vi "Gantry_GUI.vi"(0 "COMPORT":refnum<visa-resource-name>="COM5", 5 "error in (no error)":errorcluster, 7 "Antenna Select":u16(ring) items=["HOME", "TX1", "TX2", "TX3", "TX4", "TX5", "TX6", "TX7", "TX8", "TX9", "TX10", "TX11", "TX12", "RX8", "RX7", "RX6", "RX5", "RX4", "RX3", "RX2", "RX1"], 8 "EnableDriver(t)":bool=TRUE, 9 "z ref":dbl=21.0 format="%#_6f", 10 "Operation":u16(ring) items=["W/R", "RD ONLY", "WR ONLY"], 11 "Set-Z(Inches)":dbl=21.0 format="%#_6f") -> (3 "Coordinates Ref File":path=path "C:/RageATE-Tetra/Instruments/Zaber Gantry/Labview Code from Colin/Gantry/antenna_cords-4.csv", 14 "GantryGuiRefOut":refnum<vi>, 19 "error out":errorcluster)   [LabVIEW 2018]
uses:
  Initialize References/Sequence Globals.vi
  <vilib>/Utility/file.llb/Read Delimited Spreadsheet (DBL).vi
panel:
  out "stripped path":path
  in  "Exe_write":bool
  in  "Exit":bool
  out "Success?(t)":bool
  in  "Exe_ctrl":bool
  in  "Set-zMach":dbl format="%#_6f"
  out "Get-z":dbl=21.0 format="%#_6f"
  out "Get-y":dbl format="%#_13g"
  out "Get-x":dbl
  out "py path":path=path "C:/RageATE-Tetra/Instruments/Zaber Gantry/Labview Code from Colin/Gantry/Gantry.py"
  in  "Selector Control":T1(radio)
  out "comport":string="COM5"
  in  "Close Serial(t)":bool
  in  "Set-y":dbl format="%#_13g"
  in  "Set-x":dbl
  out "begin":dbl=9735.3466752 format="%_19f"
  out "List":dbl[][](array[numeric])
  # "X-Y Controls"
  # "Z Controls"
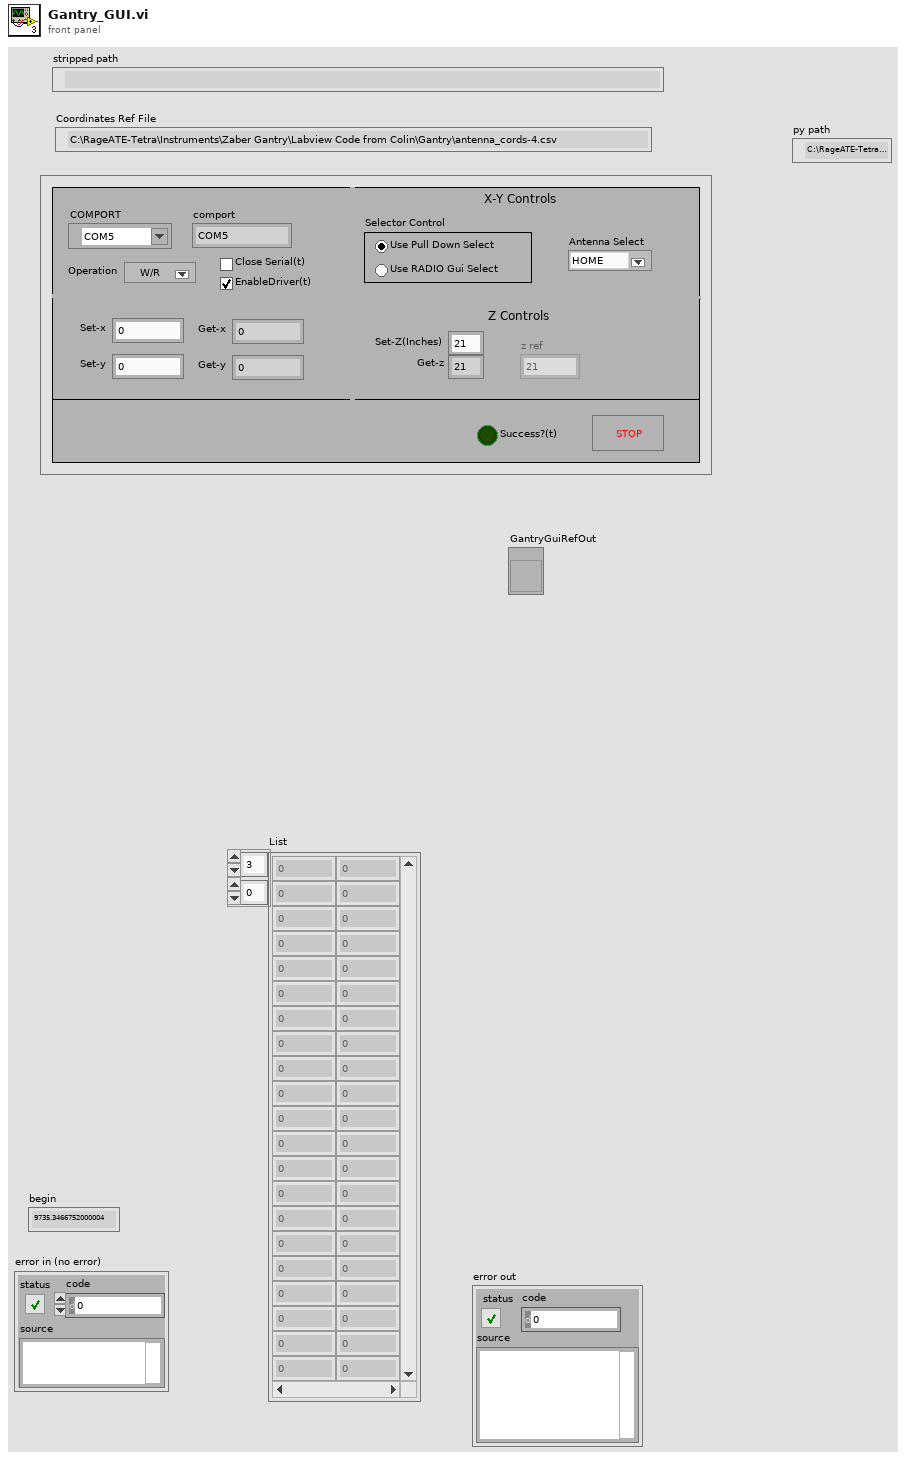
[diagram p1: front panel]
types:
  T1 = enum32{"Use Pull Down Select", "Use RADIO Gui Select"}
  T2 = enum32{"Invalid", "Standard", "Closed", "Hidden", "Minimized", "Maximized"}
  T3 = enum8{"Enabled", "Disabled", "Disabled and Grayed Out"}
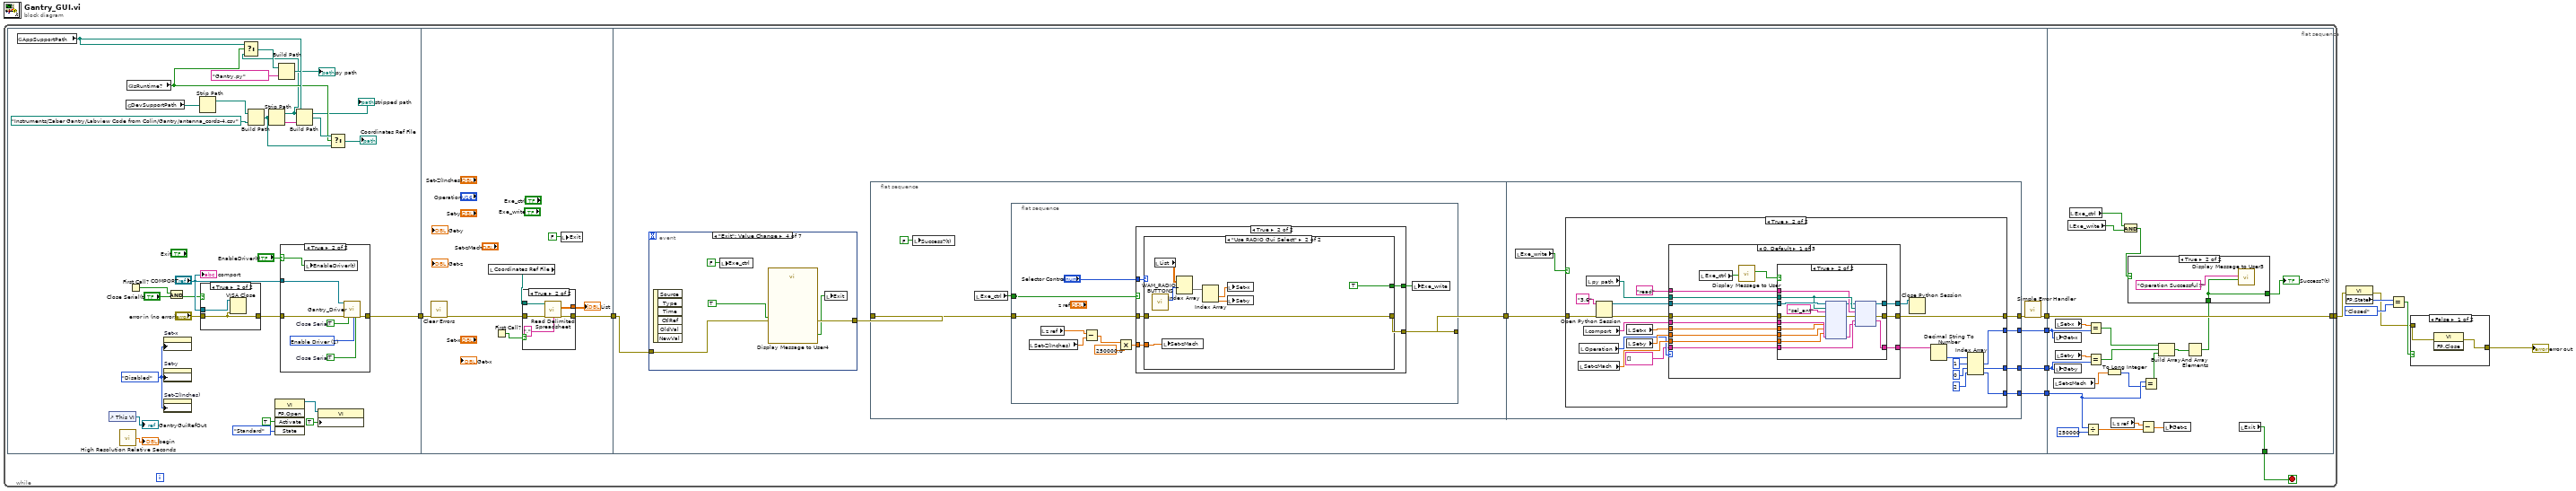
[diagram p0: block diagram]
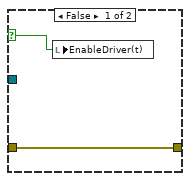
[diagram p4: hidden frame]
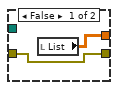
[diagram p5: hidden frame]
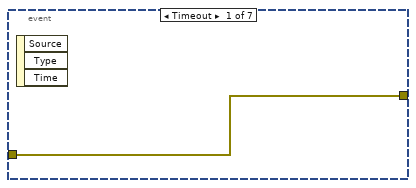
[diagram p6: hidden frame]
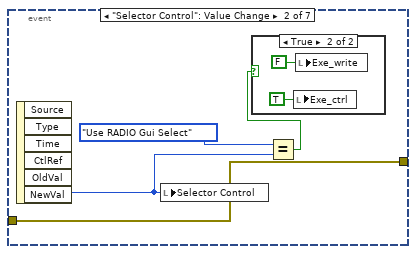
[diagram p7: hidden frame]
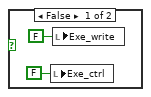
[diagram p8: hidden frame]
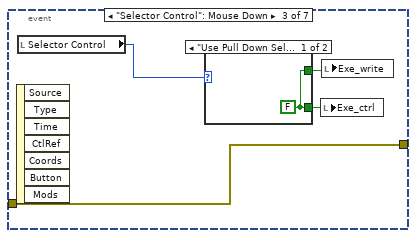
[diagram p9: hidden frame]
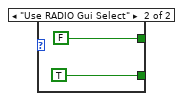
[diagram p10: hidden frame]
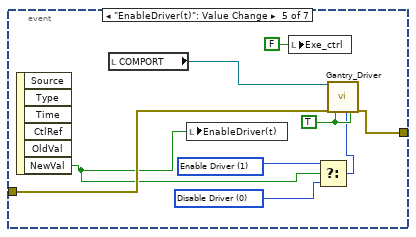
[diagram p11: hidden frame]
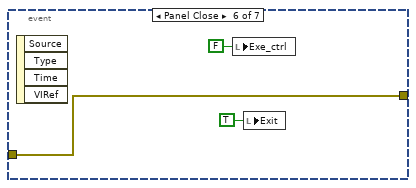
[diagram p12: hidden frame]
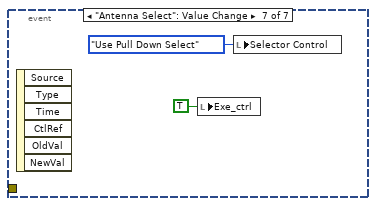
[diagram p13: hidden frame]
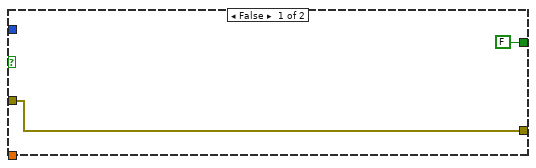
[diagram p14: hidden frame]
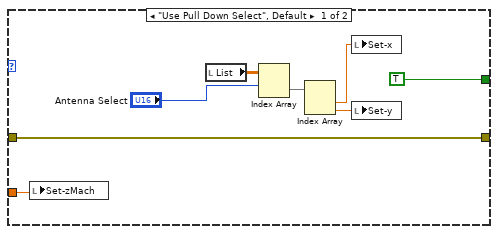
[diagram p15: hidden frame]
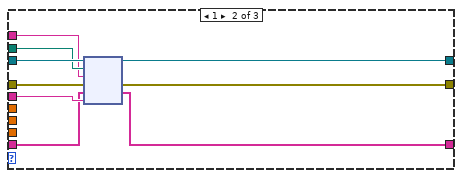
[diagram p18: hidden frame]
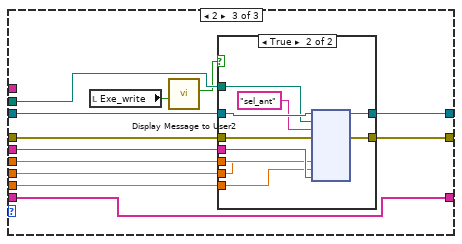
[diagram p19: hidden frame]
diagram:
  n1 = while {
    tunnel: [w8] -> w1
    stop <- w7 stop-if-true
    n2 = flat-sequence {
      tunnel: [w37] -> w14
      tunnel: w14 -> [w61]
      tunnel: [w58] -> w13
      tunnel: [w73] -> w12
      tunnel: [w76] -> w11
      tunnel: [w75] -> w10
      tunnel: [w72] -> w9
      tunnel: w13 -> [w69]
      tunnel: w12 -> [w264]
      tunnel: [w264] -> w8
      tunnel: w11 -> [w253]
      tunnel: w10 -> [w256]
      tunnel: w9 -> [w259]
      tunnel: [w248] -> w7
      frame #0 {
        w34 = T3."Disabled" ("Disabled")
        n3 = global read "Sequence Globals.vi" "AppSupportPath"() -> (w23:path)
        n4 = control-ref of="This VI"() -> (→"GantryGuiRefOut":refnum<vi>)
        n5 = call <vilib>:"High Resolution Relative Seconds.vi"() -> ("relative seconds"=→"begin":dbl)
        n6 = global read "Sequence Globals.vi" "DevSupportPath"() -> (w16:path)
        n7 = global read "Sequence Globals.vi" "IsRuntime?"() -> (w21:bool)
        n8 = First Call?() -> (First Call?: T/F=w32:bool)
        n9 = property on="Set-x" class="DigNum (strict)"("DisabledEnum"=w34) -> ()  [unwired: 2 in, 2 out]
        n10 = property on="Set-y" class="DigNum (strict)"("DisabledEnum"=w34) -> ()  [unwired: 2 in, 2 out]
        n11 = property on="Set-Z(Inches)" class="DigNum (strict)"("DisabledEnum"=w34) -> ()  [unwired: 2 in, 2 out]
        n12 = And(x=w32, y="Close Serial(t)") -> (x .and. y?=w33:bool)
        n13 = Strip Path(path=w16) -> (stripped path=w26:path)  [unwired: 1 out]
        n14 = case shown="True" w33 {
          tunnel: "error in (no error)" -> [w43 w44]
          tunnel: [w43 w44] -> w39
          tunnel: "COMPORT" -> [_ w45]
          frame False {
          }
          frame True {
            n15 = VISA Close(VISA resource name=w45, error in (no error)=w44) -> ()  [unwired: 1 out]
          }
        }
        n16 = Build Path(base path=w26, name or relative path=path "Instruments/Zaber Gantry/Labview Code from Colin/Gantry/antenna_cords-4.csv" ("file path (dialog if empty)")) -> (appended path=w25:path)
        n17 = Strip Path(path=w25) -> (stripped path=w15:path, name=w24:string)
        "stripped path" <- w15
        n18 = Select(t=w23, s=w21, f=w15) -> (s? t:f=w20:path)
        n19 = invoke class="VI" method="FP.Open"("Activate"=TRUE ("Activate?"), "State"=T2."Standard") -> (reference out=w29:refnum<vi>)  [unwired: 3 in, 4 out]
        n20 = Build Path(base path=w20, name or relative path="Gantry.py") -> (appended path=→"py path":path)
        n21 = case shown="True" "EnableDriver(t)" {
          selector: "EnableDriver(t)" -> [w46 w48]
          tunnel: "COMPORT" -> [_ w51]
          tunnel: w39 -> [w47 w54]
          tunnel: [w47 w50] -> w37
          frame False {
            n22 = local write "EnableDriver(t)"(w46) -> ()
          }
          frame True {
            w49 = TRUE  # Close Serial
            w52 = u16 1 items=["Disable Driver", "Enable Driver", "Read Driver Status"] ("Driver-Func")
            w53 = TRUE  # Close Serial
            n23 = local write "EnableDriver(t)"(w48) -> ()
            n24 = call "Gantry_Driver.vi"("VISA resource name"=w51, "error in (no error)"=w54, "Open Serial"=w53, "Driver-Func"=w52, "Close Serial"=w49) -> ("error out"=w50:errorcluster)  [unwired: 11 in, 3 out]
          }
        }
        n25 = Build Path(base path=w23, name or relative path=w24) -> (appended path=w22:path)
        n26 = property class="VI"(reference=w29, "Front Panel.IsFrontmost"=TRUE ("Front Panel Window:Is Frontmost")) -> ()  [unwired: 1 in, 2 out]
        n27 = Select(t=w22, s=w21, f=w25) -> (s? t:f=→"Coordinates Ref File":path)
        "comport" <- "COMPORT"
      }
      frame #1 {
        n28 = call <vilib>:"Clear Errors.vi"("error in (no error)"=w61) -> ("error out"=w60:errorcluster)  [unwired: 5 in, 1 out]
        n29 = local read "Coordinates Ref File"() -> (w55:path)
        n30 = First Call?() -> (First Call?: T/F=w57:bool)
        n31 = case shown="True" w57 {
          tunnel: w60 -> [w62 w68]
          tunnel: w55 -> [_ w67]
          tunnel: [w63 w65] -> w59
          tunnel: [w62 w64] -> w58
          frame False {
            n32 = local read "List"() -> (w63:dbl[][])
          }
          frame True {
            n33 = call-poly <vilib>:"Read Delimited Spreadsheet.vi"("file path (dialog if empty)"=w67, "error in (no error)"=w68, "delimiter (\\t)"="," ("delimiter (\\t)")) -> ("all rows"=w65:dbl[][], "error out"=w64:errorcluster)  [unwired: 7 in, 4 out]
          }
        }
        "List" <- w59
        n34 = local write "Exit"(FALSE ("Exit")) -> ()
      }
      frame #2 {
        n35 = event shown="[3] \"Exit\": Value Change" {
          selector: _ -> [_ _ _ _ _ _ _]
          dyn-events: _ -> [_ _ _ _ _ _ _]
          timeout: _ -> [_ _ _ _ _ _ _]
          tunnel: w69 -> [w77 w81 w89 w95 w105 w108 _]
          tunnel: [w77 w81 w89 w95 w104 w108 _] -> w70
          event Timeout {
            n36 = event-data() -> ()  [unwired: 1 in, 3 out]
          }
          event "Selector Control": Value Change {
            n37 = event-data() -> ("NewVal"=w80:T1)  [unwired: 1 in, 5 out]
            n38 = local write "Selector Control"(w80) -> ()
            n39 = Equal?(x=T1."Use RADIO Gui Select", y=w80) -> (x = y?=w78:bool)
            n40 = case shown="True" w78 {
              frame False {
                n41 = local write "Exe_ctrl"(FALSE ("Exe_ctrl")) -> ()
                n42 = local write "Exe_write"(FALSE ("Exe_write")) -> ()
              }
              frame True {
                n43 = local write "Exe_ctrl"(TRUE ("Exe_ctrl")) -> ()
                n44 = local write "Exe_write"(FALSE ("Exe_write")) -> ()
              }
            }
          }
          event "Selector Control": Mouse Down {
            n45 = event-data() -> ()  [unwired: 1 in, 7 out]
            n46 = local read "Selector Control"() -> (w88:T1)
            n47 = case shown="\"Use Pull Down Select\", Default" w88 {
              tunnel: [w90 FALSE ("Exe_write")] -> w87
              tunnel: [w90 TRUE ("Exe_ctrl")] -> w86
              frame "Use Pull Down Select", Default {
                w90 = FALSE ("Exe_ctrl")
              }
              frame "Use RADIO Gui Select" {
              }
            }
            n48 = local write "Exe_ctrl"(w86) -> ()
            n49 = local write "Exe_write"(w87) -> ()
          }
          event "Exit": Value Change {
            n50 = event-data() -> ()  [unwired: 1 in, 6 out]
            n51 = local write "Exe_ctrl"(FALSE ("Execute")) -> ()
            n52 = call "Display Message to User4"("Enable"=TRUE ("Execute")) -> ("OK"=w94:bool)  [unwired: 9 in, 1 out]
            n53 = local write "Exit"(w94) -> ()
          }
          event "EnableDriver(t)": Value Change {
            w99 = u16 0 items=["Disable Driver", "Enable Driver", "Read Driver Status"] ("Driver-Func")
            w101 = u16 1 items=["Disable Driver", "Enable Driver", "Read Driver Status"] ("Driver-Func")
            w103 = TRUE ("Open Serial")
            n54 = event-data() -> ("NewVal"=w98:bool)  [unwired: 1 in, 5 out]
            n55 = local read "COMPORT"() -> (w102:refnum<visa-resource-name>)
            n56 = local write "EnableDriver(t)"(w98) -> ()
            n57 = local write "Exe_ctrl"(FALSE ("Exe_ctrl")) -> ()
            n58 = Select(t=w101, s=w98, f=w99) -> (s? t:f=w100:u16)
            n59 = call "Gantry_Driver.vi"("VISA resource name"=w102, "error in (no error)"=w105, "Open Serial"=w103, "Driver-Func"=w100, "Close Serial"=w103) -> ("error out"=w104:errorcluster)  [unwired: 11 in, 3 out]
          }
          event Panel Close {
            n60 = event-data() -> ()  [unwired: 1 in, 4 out]
            n61 = local write "Exe_ctrl"(FALSE ("Exe_ctrl")) -> ()
            n62 = local write "Exit"(TRUE ("Exit")) -> ()
          }
          event "Antenna Select": Value Change {
            n63 = event-data() -> ()  [unwired: 1 in, 6 out]
            n64 = local write "Exe_ctrl"(TRUE ("Execute")) -> ()
            n65 = local write "Selector Control"(T1."Use Pull Down Select" ("Selector Control")) -> ()
          }
        }
        n66 = flat-sequence {
          tunnel: w70 -> [w114]
          tunnel: [w113] -> w71
          tunnel: w71 -> [w153]
          tunnel: [w152] -> w75
          tunnel: [w151] -> w76
          tunnel: [w150] -> w72
          tunnel: [w149] -> w74
          frame #0 {
            n67 = local write "Success?(t)"(FALSE ("Success?(t)")) -> ()
            n68 = local read "Exe_ctrl"() -> (w112:bool)
            n69 = flat-sequence {
              tunnel: w114 -> [w124]
              tunnel: [w123] -> w113
              tunnel: w112 -> [w116]
              frame #0 {
                n70 = local read "Set-Z(Inches)"() -> (w120:dbl)
                n71 = local read "z ref"() -> (w122:dbl)
                n72 = Subtract(x=w122, y=w120) -> (x-y=w121:dbl)
                n73 = Multiply(x=w121, y=250000.0) -> (x*y=w118:dbl)
                n74 = case shown="True" w116 {
                  tunnel: w124 -> [w125 w131]
                  tunnel: [w125 w130] -> w123
                  tunnel: w118 -> [_ w129]
                  tunnel: [FALSE ("OK") w128] -> w117
                  tunnel: "Selector Control" -> [_ w127]
                  frame False {
                  }
                  frame True {
                    n75 = case shown="\"Use RADIO Gui Select\"" w127 {
                      tunnel: w131 -> [w132 w147]
                      tunnel: [w132 w147] -> w130
                      tunnel: w129 -> [w139 w141]
                      tunnel: [TRUE ("Execute") TRUE ("Execute")] -> w128
                      frame "Use Pull Down Select", Default {
                        n76 = local write "Set-zMach"(w139) -> ()
                        n77 = local read "List"() -> (w133:dbl[][])
                        n78 = Index Array(array=w133, index (row)="Antenna Select") -> (element=w135:dbl[])  [unwired: 1 in]
                        n79 = Index Array(array=w135) -> (element #1=w136:dbl, element #2=w137:dbl)  [unwired: 2 in]
                        n80 = local write "Set-x"(w136) -> ()
                        n81 = local write "Set-y"(w137) -> ()
                      }
                      frame "Use RADIO Gui Select" {
                        n82 = call "WAM_RADIO_BUTTONS.vi"() -> ("Index out"=w145:u32)  [unwired: 11 in]
                        n83 = local read "List"() -> (w146:dbl[][])
                        n84 = local write "Set-zMach"(w141) -> ()
                        n85 = Index Array(array=w146, index (row)=w145) -> (element=w144:dbl[])  [unwired: 1 in]
                        n86 = Index Array(array=w144) -> (element #1=w143:dbl, element #2=w142:dbl)  [unwired: 2 in]
                        n87 = local write "Set-x"(w143) -> ()
                        n88 = local write "Set-y"(w142) -> ()
                      }
                    }
                  }
                }
                n89 = local write "Exe_write"(w117) -> ()
              }
            }
          }
          frame #1 {
            n90 = local read "Exe_write"() -> (w148:bool)
            n91 = case shown="True" w148 {
              tunnel: w153 -> [w154 w172]
              tunnel: [_ w171] -> w152
              tunnel: [_ w170] -> w151
              tunnel: [_ w169] -> w150
              tunnel: [w154 w168] -> w149
              frame False {
              }
              frame True {
                n92 = local read "Set-zMach"() -> (w165:dbl)
                n93 = local read "Operation"() -> (w162:u16)
                n94 = local read "comport"() -> (w163:string)
                n95 = local read "py path"() -> (w164:path)
                n96 = Open Python Session(python version="3.6" ("Python version"), 3:w172) -> (session out=w159:refnum<k35>, error out=w160:errorcluster)  [unwired: 1 in]
                n97 = local read "Set-x"() -> (w166:dbl)
                n98 = local read "Set-y"() -> (w167:dbl)
                n99 = case shown="0, Default" w162 {
                  tunnel: [w183 w216 w223] -> w158
                  tunnel: [w182 w217 w224] -> w168
                  tunnel: w164 -> [w188 w214 w228]
                  tunnel: w159 -> [w190 w215 w230]
                  tunnel: w160 -> [w189 w218 w229]
                  tunnel: w163 -> [w184 w213 w227]
                  tunnel: [w187 w212 w225] -> w161
                  tunnel: string[] [] -> [w186 w211 w225]
                  tunnel: "read" ("function name") -> [w185 w210 _]
                  tunnel: w165 -> [w181 _ w226]
                  tunnel: w166 -> [w180 _ w222]
                  tunnel: w167 -> [w179 _ w221]
                  frame 0, Default {
                    n100 = local read "Exe_ctrl"() -> (w177:bool)
                    n101 = call "Display Message to User"("Enable"=w177) -> ("OK"=w178:bool)  [unwired: 9 in, 1 out]
                    n102 = case shown="True" w178 {
                      tunnel: w190 -> [w192 w208]
                      tunnel: w189 -> [w193 w207]
                      tunnel: w188 -> [_ w206]
                      tunnel: [w191 w205] -> w187
                      tunnel: w186 -> [w191 w204]
                      tunnel: w185 -> [_ w203]
                      tunnel: w184 -> [_ w202]
                      tunnel: [w192 w200] -> w183
                      tunnel: [w193 w199] -> w182
                      tunnel: w181 -> [_ w198]
                      tunnel: w180 -> [_ w195]
                      tunnel: w179 -> [_ w194]
                      frame False {
                      }
                      frame True {
                        n103 = node(w208, w206, "sel_ant" ("function name"), w207, w195, w194, w198, w202) -> (w197:refnum<k35>, w196:errorcluster, w201:string)  [unwired: 5 in, 2 out]
                        n104 = node(w197, w206, w203, w196, w204, w201) -> (w200:refnum<k35>, w199:errorcluster, w205:string[])  [unwired: 1 in, 2 out]
                      }
                    }
                  }
                  frame 1 {
                    n105 = node(w215, w214, w210, w218, w211, w213) -> (w216:refnum<k35>, w217:errorcluster, w212:string[])  [unwired: 1 in, 2 out]
                  }
                  frame 2 {
                    n106 = local read "Exe_write"() -> (w219:bool)
                    n107 = call "Display Message to User2"("Enable"=w219) -> ("OK"=w220:bool)  [unwired: 9 in, 1 out]
                    n108 = case shown="True" w220 {
                      tunnel: w230 -> [w232 w242]
                      tunnel: w229 -> [w231 w241]
                      tunnel: w228 -> [_ w240]
                      tunnel: w227 -> [_ w239]
                      tunnel: w226 -> [_ w238]
                      tunnel: [w231 w237] -> w224
                      tunnel: [w232 w236] -> w223
                      tunnel: w222 -> [_ w235]
                      tunnel: w221 -> [_ w234]
                      frame False {
                      }
                      frame True {
                        n109 = node(w242, w240, "sel_ant" ("function name"), w241, w235, w234, w238, w239) -> (w236:refnum<k35>, w237:errorcluster)  [unwired: 6 in, 2 out]
                      }
                    }
                  }
                }
                n110 = Close Python Session(session in=w158) -> ()  [unwired: 1 in, 1 out]
                n111 = Decimal String To Number(string=w161) -> (number=w176:i32[])  [unwired: 2 in, 1 out]
                n112 = Index Array(array=w176, index #1=1 ("index"), index #2=0 ("index"), index #3=2 ("index")) -> (element #1=w171:i32, element #2=w170:i32, element #3=w169:i32)
              }
            }
          }
        }
        n113 = call <vilib>:"Simple Error Handler.vi"("error in (no error)"=w74) -> ("error out"=w73:errorcluster)  [unwired: 4 in, 4 out]
      }
      frame #3 {
        n114 = local read "Set-zMach"() -> (w258:dbl)
        n115 = local write "Get-x"(w256) -> ()
        n116 = local write "Get-y"(w253) -> ()
        n117 = local read "Set-x"() -> (w255:dbl)
        n118 = local read "Set-y"() -> (w254:dbl)
        n119 = local read "Exe_write"() -> (w246:bool)
        n120 = local read "Exe_ctrl"() -> (w247:bool)
        n121 = Divide(x=w259, y=250000) -> (x/y=w260:dbl)
        n122 = Equal?(x=w255, y=w256) -> (x = y?=w251:bool)
        n123 = Equal?(x=w254, y=w253) -> (x = y?=w250:bool)
        n124 = To Long Integer(number=w258) -> (32bit integer=w257:i32)
        n125 = local read "z ref"() -> (w261:dbl)
        n126 = And(x=w247, y=w246) -> (x .and. y?=w245:bool)
        n127 = Subtract(x=w261, y=w260) -> (x-y=w263:dbl)
        n128 = Equal?(x=w259, y=w257) -> (x = y?=w249:bool)
        n129 = Build Array(w251, w250, w249) -> (w252:bool[])
        n130 = local write "Get-z"(w263) -> ()
        n131 = And Array Elements(Boolean array=w252) -> (logical AND=w244:bool)
        n132 = case shown="True" w245 {
          tunnel: w244 -> [_ w266]
          tunnel: [FALSE w266] -> w243
          frame False {
          }
          frame True {
            n133 = call "Display Message to User3"("Enable"=w266, "Message"="Operation Successful!!") -> ()  [unwired: 8 in, 2 out]
          }
        }
        "Success?(t)" <- w243
        n134 = local read "Exit"() -> (w248:bool)
      }
    }
  }
  n135 = property class="VI"(error in=w1) -> (error out=w2:errorcluster, "FP.State"=w5:T2)  [unwired: 1 in, 1 out]
  n136 = Equal?(x=w5, y=T2."Closed") -> (x = y?=w3:bool)
  n137 = case shown="False" w3 {
    tunnel: w2 -> [w269 w270]
    tunnel: [w268 w270] -> w6
    frame False {
      n138 = invoke class="VI" method="FP.Close"(error in=w269) -> (error out=w268:errorcluster)  [unwired: 2 in, 2 out]
    }
    frame True {
    }
  }
  "error out" <- w6
